vi "GetChannelFromSignal.vi"(8 "Error in":errorcluster, 10 "Signal":refnum<k24>, 11 "DevicesAndSignals":T1) -> (0 "Error out":errorcluster, 2 "Channel":refnum<k24>, 3 "DevicesAndSignals":T1)   [LabVIEW 2016]
doc: "Finds the channel to which the given signal belongs.\n\nSignal: Signal to check to which channel it belongs\nChannel: The channel to which the signal belongs"
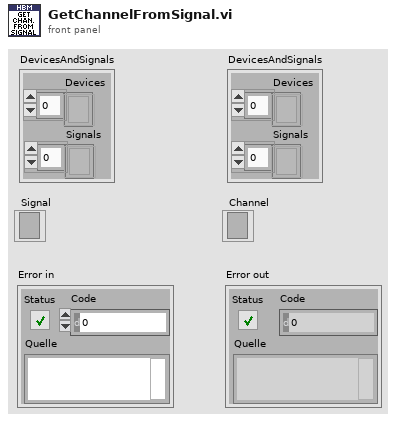
[diagram p1: front panel]
types:
  T1 = cluster{"Devices":refnum<k24>[], "Signals":refnum<k24>[]}
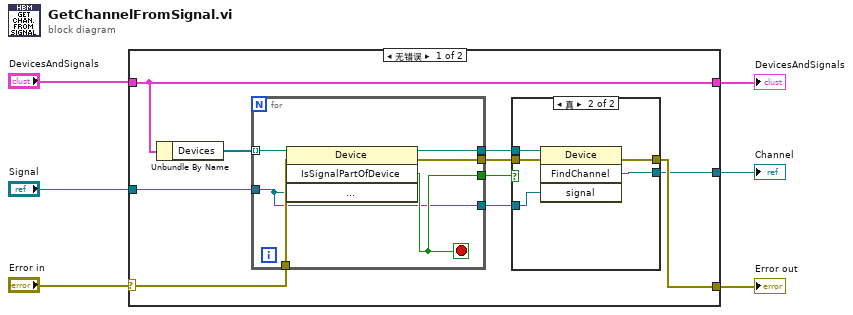
[diagram p0: block diagram]
diagram:
  n1 = case shown="无错误" "Error in" {
    selector: "Error in" -> [w11 w30]
    tunnel: [w8 w30] -> w6
    tunnel: [w16 w29] -> w3
    tunnel: "DevicesAndSignals" -> [w16 w29]
    tunnel: "Signal" -> [w14 _]
    tunnel: [w7 _] -> w1
    frame No Error {
      n2 = Unbundle By Name(w16) -> ("Devices"=w15:refnum<k24>[])
      n3 = for {
        tunnel: w15 -> [w28] mode=indexing
        tunnel: w14 -> [w23]
        tunnel: [w27] -> w13
        tunnel: [w26] -> w12
        tunnel: w11 -> [w25]
        tunnel: [w24] -> w9
        tunnel: [w23] -> w10
        stop <- w27 stop-if-true
        n4 = invoke on="Methodenknoten" class="Device" method="IsSignalPartOfDevice"(reference=w28, error in=w25, "signalToCheck"=w23) -> (reference out=w26:refnum<k24>, error out=w24:errorcluster, "IsSignalPartOfDevice"=w27:bool)  [unwired: 1 in, 1 out]
      }
      n5 = case shown="真" w13 {
        tunnel: w12 -> [_ w22]
        tunnel: w10 -> [_ w21]
        tunnel: w9 -> [w17 w20]
        tunnel: [w17 w19] -> w8
        tunnel: [_ w18] -> w7
        frame False {
        }
        frame True {
          n6 = invoke on="Methodenknoten" class="Device" method="FindChannel"(reference=w22, error in=w20, "signal"=w21) -> (error out=w19:errorcluster, "FindChannel"=w18:refnum<k24>)  [unwired: 1 in, 2 out]
        }
      }
    }
    frame Error {
    }
  }
  "Error out" <- w6
  "DevicesAndSignals" <- w3
  "Channel" <- w1
